vi "parse_config_list.vi"(11 "String":string) -> (2 "Values":dbl[](array[numeric]), 3 "Names":string[](array[string]))   [LabVIEW 2025, in "LabJackEKG.lvlib"]
uses:
  LabJackEKG.lvlib
  <vilib>/Utility/error.llb/Trim Whitespace One-Sided.vi
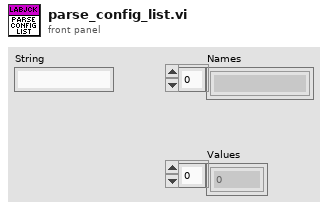
[diagram p1: front panel]
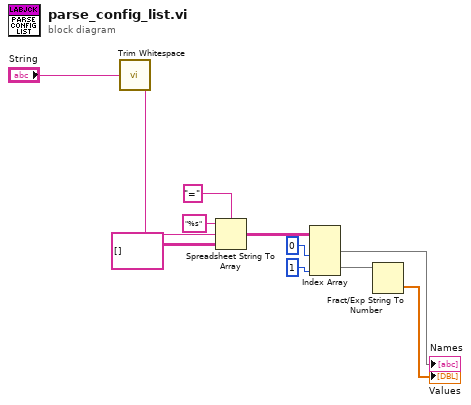
[diagram p0: block diagram]
diagram:
  n1 = call <vilib>:"Trim Whitespace.vi"("string"="String") -> ("trimmed string"=w11:string)  [unwired: 1 in]
  n2 = Spreadsheet String To Array(delimiter (Tab)="=", format string="%s", spreadsheet string=w11, array type (2D Dbl)=string[][] []) -> (array=w4:string[][])
  n3 = Index Array(array=w4, index (col) #1=0 ("disabled index (col)"), index (col) #2=1 ("index (col)")) -> (element #1=→"Names":string[], element #2=w7:string[])  [unwired: 2 in]
  n4 = Fract/Exp String To Number(string=w7) -> (number=→"Values":dbl[])  [unwired: 3 in, 1 out]
